vi "Update Time.vi"(0 "reference in":refnum<class "Timer.lvclass">, 3 "Timer Time (ms)":u32, 5 "error in (no error)":errorcluster) -> (14 "reference out":refnum<class "Timer.lvclass">, 19 "error out":errorcluster)   [LabVIEW 2017, in "Timer.lvclass"]
uses:
  Timer.lvclass
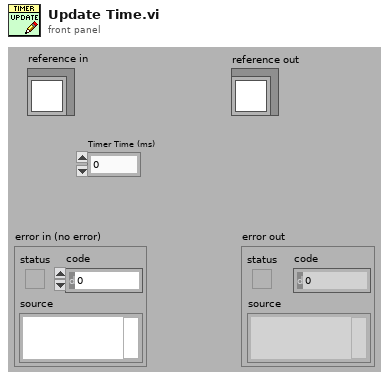
[diagram p1: front panel]
types:
  T1 = typedef "Timer.lvclass/ObjectAttributes.ctl" = cluster{"Timer is Timing":bool, "Timer Time (ms)":u32, "Timer VI Reference":refnum<vi>}
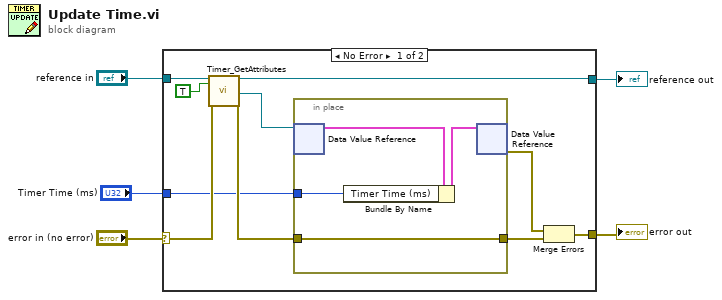
[diagram p0: block diagram]
diagram:
  n1 = case shown="No Error" "error in (no error)" {
    selector: "error in (no error)" -> [w12 w21]
    tunnel: [w14 w21] -> w4
    tunnel: [w10 w20] -> w2
    tunnel: "reference in" -> [w13 w20]
    tunnel: "Timer Time (ms)" -> [w6 _]
    frame No Error {
      n2 = call "Timer_GetAttributes.vi"("reference in"=w13, "OnlyGetDvrReference(False)"=TRUE, "error in (no error)"=w12) -> ("reference out"=w10:refnum<class "Timer.lvclass">, "DataRef"=w11:refnum<data-value>, "error out"=w8:errorcluster)  [unwired: 13 in, 1 out]
      n3 = in-place {
        in-place-border: w8 -> [w18]
        in-place-border: [w18] -> w7
        in-place-border: w6 -> [w16]
        n4 = in-place-dvr #1(w11) -> (w17:T1)  [unwired: 1 out]
        n5 = Bundle By Name(cluster=w17, "Timer Time (ms)"=w16) -> (w19:T1)
        n6 = in-place-dvr #1(w19) -> (w15:errorcluster)  [unwired: 1 out]
      }
      n7 = Merge Errors(w15, w7) -> (w14:errorcluster)
    }
    frame Error {
    }
  }
  "error out" <- w4
  "reference out" <- w2
